vi "Read Element of Array of ccd.vi"(8 "error in (no error)":errorcluster, 10 "index":i32, 11 "CCD monitor in":refnum<class "CCD monitor.lvclass">) -> (0 "error out":errorcluster, 2 "Hardware.lvlib:CCD.lvlib:CCD.lvclass":refnum<class "CCD.lvclass">, 3 "CCD monitor out":refnum<class "CCD monitor.lvclass">)   [LabVIEW 2016, in "Hardware.lvlib" / "CCD monitor.lvlib" / "CCD monitor.lvclass"]
uses:
  <userlib>/Common Components/Hardware/Abstract System/Monitor/CCD monitor.lvclass
  <userlib>/Common Components/Hardware/CCD/CCD/CCD.lvclass
  <userlib>/Common Components/Hardware/Abstract System/Monitor/CCD monitor.lvclass/CCD monitor.ctl
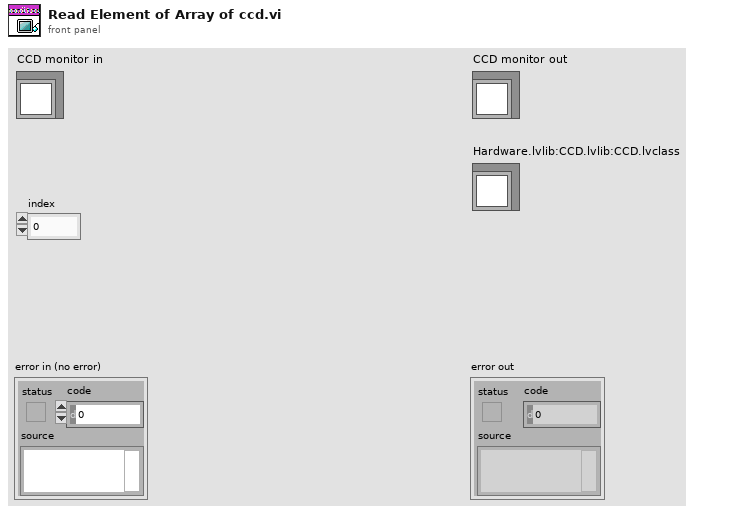
[diagram p1: front panel]
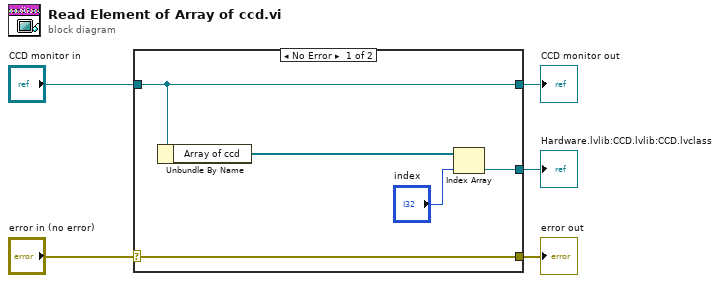
[diagram p0: block diagram]
diagram:
  n1 = case shown="No Error" "error in (no error)" {
    selector: "error in (no error)" -> [w10 w11]
    tunnel: [w10 w11] -> w4
    tunnel: [w9 w12] -> w2
    tunnel: "CCD monitor in" -> [w9 w12]
    tunnel: [w6 _] -> w1
    frame No Error {
      n2 = Unbundle By Name(w9) -> ("Array of ccd"=w8:refnum<class "CCD.lvclass">[])
      n3 = Index Array(array=w8, index="index") -> (element=w6:refnum<class "CCD.lvclass">)
    }
    frame Error {
    }
  }
  "error out" <- w4
  "CCD monitor out" <- w2
  "Hardware.lvlib:CCD.lvlib:CCD.lvclass" <- w1
